vi "Periodic Tasks.vi"(8 "error in":errorcluster) -> ()   [LabVIEW 2015]
doc: "This VI runs in parallel to other tasks. It can contain as many user-defined periodic loops as you need. These can carry out PID or other sorts of timed response."
uses:
  <vilib>/Rock Robotics/WPI/DriverStation/WPI_DriverStationRobotMode2.ctl
  <vilib>/Rock Robotics/WPI/Utilities/WPI_GetSetVariantRefNum.vi
  Utilities/MotorPositionGlobals.vi
  Utilities/VisionGlobals.vi
  Utilities/ShiftGlobals.vi
  Utilities/GeneralGlobals.vi
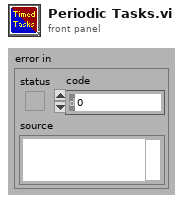
[diagram p1: front panel]
types:
  T1 = typedef "WPI_DriverStationRobotMode2.ctl" = enum16{"Autonomous Disabled", "Autonomous Enabled", "Teleop Disabled", "Teleop Enabled", "Disconnected", "Finish", "Test Disabled", "Test Enabled", "Emergency Stopped"}
  T2 = typedef "WPI_JoystickDevRef.ctl" = cluster{"Device":T3}
  T3 = typedef "WPI_JoystickDeviceEnum.ctl" = enum16{"USB 0", "USB 1", "USB 2", "USB 3", "USB 4", "USB 5"}
  T4 = typedef "WPI_DigitalOutputDevRef.ctl" = cluster{"DIO Channel":T5, "DevStatus":errorcluster}
  T5 = typedef "FPGA_DIOChannel.ctl" = enum8{"DIO 0", "DIO 1", "DIO 2", "DIO 3", "DIO 4", "DIO 5", "DIO 6", "DIO 7", "DIO 8", "DIO 9", "DIO MXP 0", "DIO MXP 1", "DIO MXP 2", "DIO MXP 3", "DIO MXP 4", "DIO MXP 5", "DIO MXP 6", "DIO MXP 7", "DIO MXP 8", "DIO MXP 9", "DIO MXP 10", "DIO MXP 11", "DIO MXP 12", "DIO MXP 13", "DIO MXP 14", "DIO MXP 15", "Invalid"}
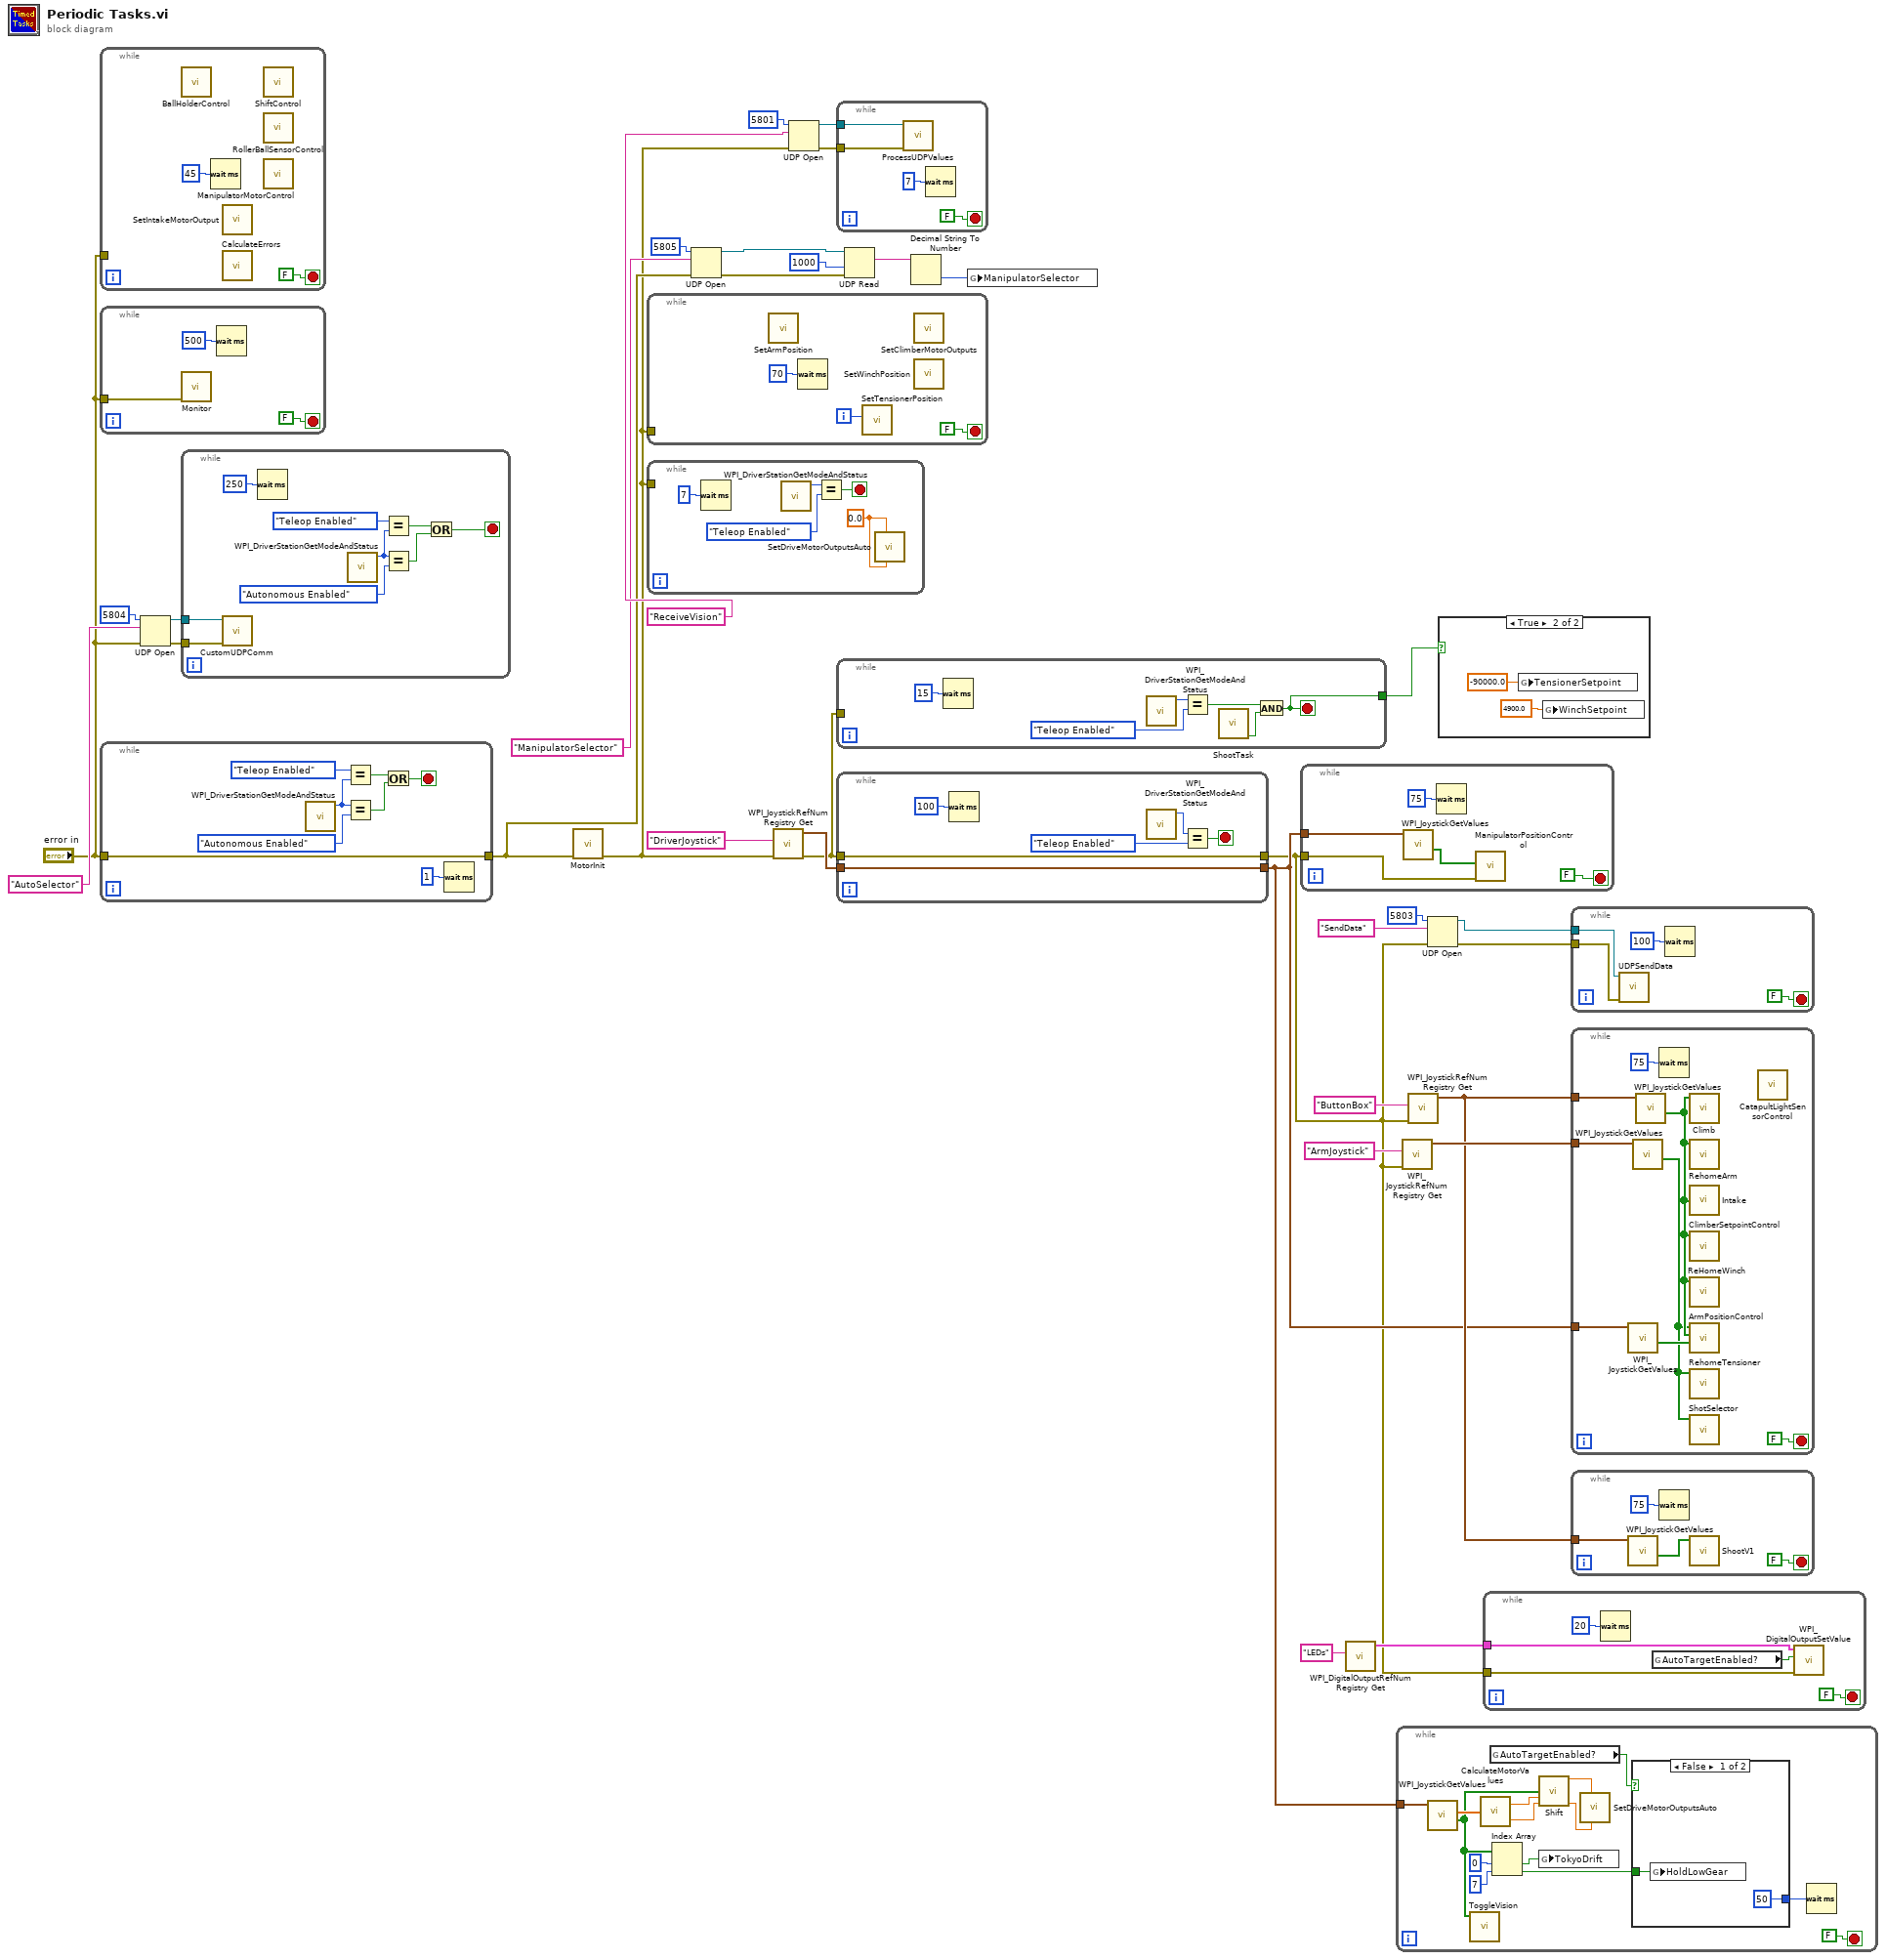
[diagram p0: block diagram]
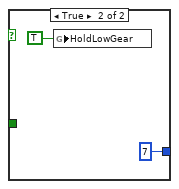
[diagram p3: hidden frame]
diagram:
  n1 = while {
    tunnel: "error in" -> [_]
    stop <- FALSE stop-if-true
    n2 = call "BallHolderControl.vi"() -> ()  [unwired: 12 in]
    n3 = Wait (ms)(milliseconds to wait=u32 45) -> ()  [unwired: 1 out]
    n4 = call "SetIntakeMotorOutput.vi"() -> ()  [unwired: 3 in]
    n5 = call "CalculateErrors.vi"() -> ()  [unwired: 12 in]
    n6 = call "ShiftControl.vi"() -> ()  [unwired: 12 in]
    n7 = call "RollerBallSensorControl.vi"() -> ()  [unwired: 12 in]
    n8 = call "ManipulatorMotorControl.vi"() -> ()  [unwired: 12 in]
  }
  n9 = while {
    tunnel: "error in" -> [w37]
    stop <- FALSE stop-if-true
    n10 = call "Monitor.vi"("error in (no error)"=w37) -> ()  [unwired: 11 in]
    n11 = Wait (ms)(milliseconds to wait=u32 500) -> ()  [unwired: 1 out]
  }
  n12 = while {
    tunnel: "error in" -> [w43]
    tunnel: [w43] -> w10
    stop <- w41 stop-if-true
    n13 = call <vilib>:"WPI_DriverStationGetModeAndStatus.vi"() -> ("Robot Mode"=w46:T1)  [unwired: 10 in, 1 out]
    n14 = Equal?(x=WPI_DriverStationRobotMode2."Teleop Enabled" ("Robot Mode"), y=w46) -> (x = y?=w44:bool)
    n15 = Equal?(x=w46, y=WPI_DriverStationRobotMode2."Autonomous Enabled" ("Robot Mode")) -> (x = y?=w40:bool)
    n16 = Or(x=w44, y=w40) -> (x .or. y?=w41:bool)
    n17 = Wait (ms)(milliseconds to wait=u32 1) -> ()  [unwired: 1 out]
  }
  n18 = UDP Open(8:"error in", 10:"AutoSelector" ("service name"), 11:u16 5804 ("port")) -> (port=w30:refnum<k16>, 0:w29:errorcluster)  [unwired: 2 in, 1 out]
  n19 = while {
    tunnel: w30 -> [w55]
    tunnel: w29 -> [w54]
    stop <- w48 stop-if-true
    n20 = call "CustomUDPComm.vi"("error in (no error)"=w54, "connection ID"=w55) -> ()  [unwired: 9 in, 1 out]
    n21 = Wait (ms)(milliseconds to wait=u32 250) -> ()  [unwired: 1 out]
    n22 = call <vilib>:"WPI_DriverStationGetModeAndStatus.vi"() -> ("Robot Mode"=w52:T1)  [unwired: 10 in, 1 out]
    n23 = Equal?(x=WPI_DriverStationRobotMode2."Teleop Enabled" ("Robot Mode"), y=w52) -> (x = y?=w50:bool)
    n24 = Equal?(x=w52, y=WPI_DriverStationRobotMode2."Autonomous Enabled" ("Robot Mode")) -> (x = y?=w49:bool)
    n25 = Or(x=w50, y=w49) -> (x .or. y?=w48:bool)
  }
  n26 = call "MotorInit.vi"("error in (no error)"=w10) -> ("error out"=w4:errorcluster)  [unwired: 10 in]
  n27 = while {
    tunnel: w4 -> [_]
    i -> [w57]
    stop <- FALSE stop-if-true
    n28 = call "SetArmPosition.vi"() -> ()  [unwired: 12 in]
    n29 = Wait (ms)(milliseconds to wait=u32 70) -> ()  [unwired: 1 out]
    n30 = call "SetTensionerPosition.vi"("LoopCount"=w57) -> ()  [unwired: 11 in]
    n31 = call "SetClimberMotorOutputs.vi"() -> ()  [unwired: 12 in]
    n32 = call "SetWinchPosition.vi"() -> ()  [unwired: 12 in]
  }
  n33 = while {
    tunnel: w4 -> [_]
    stop <- w62 stop-if-true
    w60 = 0.0 ("LeftMotorOutput")
    n34 = Wait (ms)(milliseconds to wait=u32 7) -> ()  [unwired: 1 out]
    n35 = call <vilib>:"WPI_DriverStationGetModeAndStatus.vi"() -> ("Robot Mode"=w64:T1)  [unwired: 10 in, 1 out]
    n36 = Equal?(x=w64, y=WPI_DriverStationRobotMode2."Teleop Enabled" ("Robot Mode")) -> (x = y?=w62:bool)
    n37 = call "SetDriveMotorOutputsAuto.vi"("RightMotorOutput"=w60, "LeftMotorOutput"=w60) -> ()  [unwired: 5 in]
  }
  n38 = UDP Open(8:w10, 10:"ManipulatorSelector" ("service name"), 11:u16 5805 ("port")) -> (port=w12:refnum<k16>, 0:w13:errorcluster)  [unwired: 2 in, 1 out]
  n39 = call <vilib>:"WPI_JoystickRefNum Registry Get.vi"("error in (no error)"=w4, "refnum name"="DriverJoystick") -> ("error out"=w3:errorcluster, "JoystickDevRef"=w28:T2)  [unwired: 8 in]
  n40 = UDP Open(8:w4, 10:"ReceiveVision" ("service name"), 11:u16 5801 ("port")) -> (port=w25:refnum<k16>, 0:w24:errorcluster)  [unwired: 2 in, 1 out]
  n41 = while {
    tunnel: w25 -> [w66]
    tunnel: w24 -> [w65]
    stop <- FALSE stop-if-true
    n42 = call "ProcessUDPValues.vi"("error in (no error)"=w65, "connection ID"=w66) -> ()  [unwired: 10 in]
    n43 = Wait (ms)(milliseconds to wait=u32 7) -> ()  [unwired: 1 out]
  }
  n44 = while {
    tunnel: w3 -> [_]
    tunnel: [w69] -> w1
    stop <- w69 stop-if-true
    n45 = Wait (ms)(milliseconds to wait=u32 15) -> ()  [unwired: 1 out]
    n46 = call <vilib>:"WPI_DriverStationGetModeAndStatus.vi"() -> ("Robot Mode"=w74:T1)  [unwired: 10 in, 1 out]
    n47 = Equal?(x=w74, y=WPI_DriverStationRobotMode2."Teleop Enabled" ("Robot Mode")) -> (x = y?=w71:bool)
    n48 = call "ShootTask.vi"() -> ("DoneReloading"=w70:bool)  [unwired: 11 in]
    n49 = And(x=w71, y=w70) -> (x .and. y?=w69:bool)
  }
  n50 = while {
    tunnel: w28 -> [w80]
    tunnel: [w80] -> w5
    tunnel: w3 -> [w75]
    tunnel: [w75] -> w2
    stop <- w77 stop-if-true
    n51 = Wait (ms)(milliseconds to wait=u32 100) -> ()  [unwired: 1 out]
    n52 = call <vilib>:"WPI_DriverStationGetModeAndStatus.vi"() -> ("Robot Mode"=w79:T1)  [unwired: 10 in, 1 out]
    n53 = Equal?(x=w79, y=WPI_DriverStationRobotMode2."Teleop Enabled" ("Robot Mode")) -> (x = y?=w77:bool)
  }
  n54 = UDP Read(connection ID=w12, timeout ms (25000)=1000, 8:w13) -> (data out=w14:string)  [unwired: 1 in, 4 out]
  n55 = Decimal String To Number(string=w14) -> (number=w6:i32)  [unwired: 2 in, 1 out]
  n56 = global write "GeneralGlobals.vi" "ManipulatorSelector"(w6) -> ()
  n57 = while {
    tunnel: w5 -> [w83]
    tunnel: w2 -> [w82]
    stop <- FALSE stop-if-true
    n58 = call <vilib>:"WPI_JoystickGetValues.vi"("JoystickDevRef"=w83) -> ("Buttons"=w81:bool[])  [unwired: 6 in, 4 out]
    n59 = Wait (ms)(milliseconds to wait=u32 75) -> ()  [unwired: 1 out]
    n60 = call "ManipulatorPositionControl.vi"("error in (no error)"=w82, "ButtonArray"=w81) -> ()  [unwired: 10 in]
  }
  n61 = call <vilib>:"WPI_DigitalOutputRefNum Registry Get.vi"("refnum name"="LEDs") -> ("DigitalOutputDevRef"=w9:T4)  [unwired: 9 in, 1 out]
  n62 = while {
    tunnel: w5 -> [w94]
    stop <- FALSE stop-if-true
    n63 = call <vilib>:"WPI_JoystickGetValues.vi"("JoystickDevRef"=w94) -> ("Buttons"=w92:bool[], "Axes"=w93:dbl[])  [unwired: 6 in, 3 out]
    n64 = call "ToggleVision.vi"("ButtonArray"=w92) -> ()  [unwired: 11 in]
    n65 = call "CalculateMotorValues.vi"("Axes"=w93) -> ("LeftSideMotors"=w97:dbl, "RightSideMotors"=w98:dbl)
    n66 = global read "VisionGlobals.vi" "AutoTargetEnabled?"() -> (w95:bool)
    n67 = Index Array(array=w92, index #1=0 ("index"), index #2=7 ("index")) -> (element #1=w91:bool, element #2=w90:bool)
    n68 = call "Shift.vi"("Buttons"=w92, "CalculatedLeftMotorOutput"=w97, "CalculatedRightMotorOutput"=w98) -> ("LeftMotorOutput"=w87:dbl, "RightMotorOutput"=w86:dbl)  [unwired: 11 in]
    n69 = global write "MotorPositionGlobals.vi" "TokyoDrift"(w91) -> ()
    n70 = call "SetDriveMotorOutputsAuto.vi"("RightMotorOutput"=w86, "LeftMotorOutput"=w87) -> ()  [unwired: 5 in]
    n71 = case shown="False" w95 {
      tunnel: [u32 50 ("milliseconds to wait") u32 7 ("milliseconds to wait")] -> w96
      tunnel: w90 -> [w100 _]
      frame False {
        n72 = global write "ShiftGlobals.vi" "HoldLowGear"(w100) -> ()
      }
      frame True {
        n73 = global write "ShiftGlobals.vi" "HoldLowGear"(TRUE ("HoldLowGear")) -> ()
      }
    }
    n74 = Wait (ms)(milliseconds to wait=w96) -> ()  [unwired: 1 out]
  }
  n75 = call <vilib>:"WPI_JoystickRefNum Registry Get.vi"("error in (no error)"=w2, "refnum name"="ArmJoystick") -> ("JoystickDevRef"=w23:T2)  [unwired: 8 in, 1 out]
  n76 = call <vilib>:"WPI_JoystickRefNum Registry Get.vi"("error in (no error)"=w2, "refnum name"="ButtonBox") -> ("JoystickDevRef"=w7:T2)  [unwired: 8 in, 1 out]
  n77 = UDP Open(8:w2, 10:"SendData" ("service name"), 11:u16 5803 ("port")) -> (port=w19:refnum<k16>, 0:w18:errorcluster)  [unwired: 2 in, 1 out]
  n78 = case shown="True" w1 {
    frame False {
    }
    frame True {
      n79 = global write "MotorPositionGlobals.vi" "TensionerSetpoint"(-90000.0 ("TensionerSetpoint")) -> ()
      n80 = global write "MotorPositionGlobals.vi" "WinchSetpoint"(4900.0 ("WinchSetpoint")) -> ()
    }
  }
  n81 = while {
    tunnel: w9 -> [w108]
    tunnel: w2 -> [w106]
    stop <- FALSE stop-if-true
    n82 = Wait (ms)(milliseconds to wait=u32 20) -> ()  [unwired: 1 out]
    n83 = global read "VisionGlobals.vi" "AutoTargetEnabled?"() -> (w109:bool)
    n84 = call <vilib>:"WPI_DigitalOutputSetValue.vi"("error in (no error)"=w106, "Value"=w109, "DigitalOutputDevRef"=w108) -> ()  [unwired: 7 in, 2 out]
  }
  n85 = while {
    tunnel: w19 -> [w112]
    tunnel: w18 -> [w111]
    stop <- FALSE stop-if-true
    n86 = call "UDPSendData.vi"("error in (no error)"=w111, "connection ID"=w112) -> ()  [unwired: 10 in]
    n87 = Wait (ms)(milliseconds to wait=u32 100) -> ()  [unwired: 1 out]
  }
  n88 = while {
    tunnel: w23 -> [w121]
    tunnel: w7 -> [w119]
    tunnel: w5 -> [w118]
    stop <- FALSE stop-if-true
    n89 = call <vilib>:"WPI_JoystickGetValues.vi"("JoystickDevRef"=w118) -> ("Buttons"=w117:bool[])  [unwired: 6 in, 4 out]
    n90 = call <vilib>:"WPI_JoystickGetValues.vi"("JoystickDevRef"=w121) -> ("Buttons"=w115:bool[])  [unwired: 6 in, 4 out]
    n91 = call <vilib>:"WPI_JoystickGetValues.vi"("JoystickDevRef"=w119) -> ("Buttons"=w116:bool[])  [unwired: 6 in, 4 out]
    n92 = Wait (ms)(milliseconds to wait=u32 75) -> ()  [unwired: 1 out]
    n93 = call "Climb.vi"("Buttons"=w116) -> ()  [unwired: 11 in]
    n94 = call "RehomeArm.vi"("Buttons"=w116) -> ()  [unwired: 11 in]
    n95 = call "Intake.vi"("Buttons"=w116) -> ()  [unwired: 1 in]
    n96 = call "ClimberSetpointControl.vi"("Buttons"=w116) -> ()  [unwired: 11 in]
    n97 = call "ReHomeWinch.vi"("Buttons"=w116) -> ()  [unwired: 11 in]
    n98 = call "ArmPositionControl.vi"("DriverJoystickButtons"=w117, "ButtonBox2"=w116, "Buttons"=w115) -> ()  [unwired: 9 in]
    n99 = call "RehomeTensioner.vi"("Buttons"=w115) -> ()  [unwired: 11 in]
    n100 = call "ShotSelector.vi"("Buttons"=w115) -> ()  [unwired: 11 in]
    n101 = call "CatapultLightSensorControl.vi"() -> ()  [unwired: 12 in]
  }
  n102 = while {
    tunnel: w7 -> [w124]
    stop <- FALSE stop-if-true
    n103 = call <vilib>:"WPI_JoystickGetValues.vi"("JoystickDevRef"=w124) -> ("Buttons"=w123:bool[])  [unwired: 6 in, 4 out]
    n104 = Wait (ms)(milliseconds to wait=u32 75) -> ()  [unwired: 1 out]
    n105 = call "ShootV1.vi"("Butons"=w123) -> ()  [unwired: 11 in]
  }
